vi "BL_TestCommSpeed.vi"(8 "error in (no error)":errorcluster, 10 "Channel":u8 max=15, 11 "Potentiostat Galvanostat in":refnum<class "Potentiostat Galvanostat.lvclass">) -> (0 "error out":errorcluster, 1 "Channel Speed (ms)":i32, 2 "Device Speed (ms)":i32, 3 "Potentiostat Galvanostat out":refnum<class "Potentiostat Galvanostat.lvclass">)   [LabVIEW 2018, in "Potentiostat Galvanostat.lvclass"]
doc: "This function tests the communication speed between the library and the selected channel. \nNOTE: This function is for advanced user only."
uses:
  Potentiostat Galvanostat.lvclass
  Potentiostat Galvanostat.lvclass/Potentiostat Galvanostat.ctl
  BL_GetErrorMsg.vi
  <vilib>/Utility/error.llb/Error Cluster From Error Code.vi
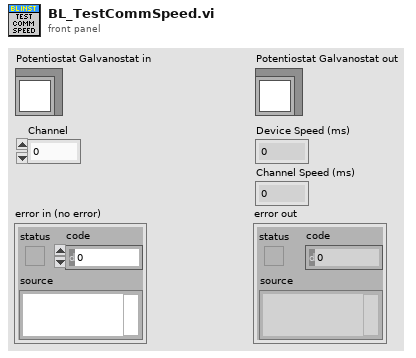
[diagram p1: front panel]
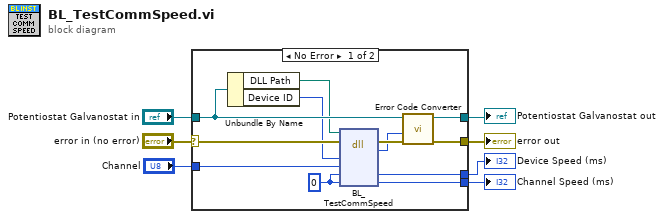
[diagram p0: block diagram]
diagram:
  n1 = case shown="No Error" "error in (no error)" {
    selector: "error in (no error)" -> [w16 w21]
    tunnel: [w19 w21] -> w6
    tunnel: [w18 w20] -> w4
    tunnel: "Potentiostat Galvanostat in" -> [w17 w20]
    tunnel: "Channel" -> [w11 _]
    tunnel: [w9 _] -> w2
    tunnel: [w8 _] -> w1
    frame No Error {
      w10 = 0 ("Device Speed (ms)")
      n2 = Unbundle By Name(w17) -> ("DLL Path"=w14:path, "Device ID"=w12:i32)
      n3 = dll-call lib="C:/Program Files (x86)/National Instruments/LabVIEW 2018/user.lib/EClib/EClib.*" fn="BL_TestCommSpeed"(path in=w14, error in=w16, "Device ID"=w12, "Channel"=w11, "Device Speed (ms)"=w10, "Channel Speed (ms)"=w10) -> (error out=w15:errorcluster, "Error Code"=w13:i32, "Device Speed (ms)"=w9:i32, "Channel Speed (ms)"=w8:i32)  [unwired: 3 in, 1 out]
      n4 = call "Error Code Converter.vi"("error in (no error)"=w15, "Error Code"=w13, "Potentiostat Galvanostat in"=w17) -> ("error out"=w19:errorcluster, "Potentiostat Galvanostat out"=w18:refnum<class "Potentiostat Galvanostat.lvclass">)  [unwired: 7 in]
    }
    frame Error {
    }
  }
  "error out" <- w6
  "Potentiostat Galvanostat out" <- w4
  "Device Speed (ms)" <- w2
  "Channel Speed (ms)" <- w1
